vi "3 Axis Step Move.vi"(0 "Reference In":refnum<class "_Controller.lvclass">, 3 "Move":bool, 7 "Error In":errorcluster, 8 "X Steps":string="0", 9 "Direction X":bool=TRUE, 10 "Y Steps":string="0", 11 "Direction Y":bool=TRUE, 12 "Z Steps":string="0", 13 "Direcition Z":bool=TRUE) -> (20 "Reference Out":refnum<class "_Controller.lvclass">, 27 "Error Out":errorcluster)   [LabVIEW 2020]
doc: "Sends commands to the machine to move it in all 3 axes. Default values set at 0 steps, so can be used to only move in 2/3 axes or 1/3 axes. Made up of a series of sub_vi's (in a case structure) to move it in all 3 axis's with their respective inputs being the number of steps it needs to move as well as the direction that motor needs to move in. \n\nArgs:\n\nReference In: Incoming communication (reference) between LabView and the scanning rig controller\nError In: Checks for any errors with the incoming communication (reference)\nX Steps: Number of steps in the X direction\nY Steps: Number of steps in the Y direction\nZ Steps: Number of steps in the Z direction\nDirection X: Direction that the X stepper motor needs to move in\nDirection Y: Direction that the Y stepper motor needs to move in\nDIrection Z: Direction that the Z stepper motor needs to move in\n\nReturns:\n\nReference Out: Output communnication (reference) between LabView and controller\nError Out: Checks for any error with output communication (reference)"
uses:
  <instrlib>/Arcus Ethernet Driver 1.0.0/ArcusEthernetComm/classes/Controller/_Controller.lvclass
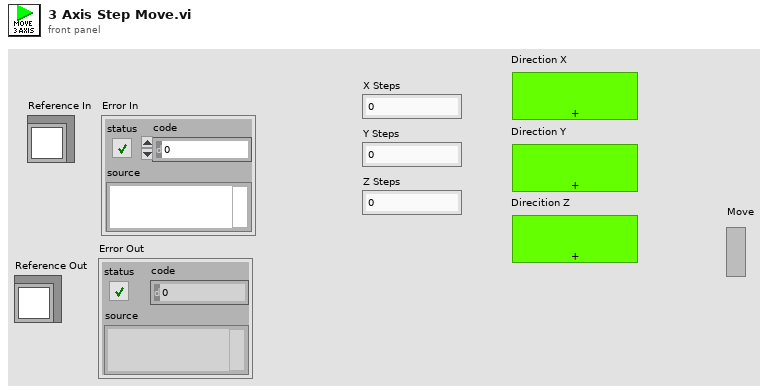
[diagram p1: front panel]
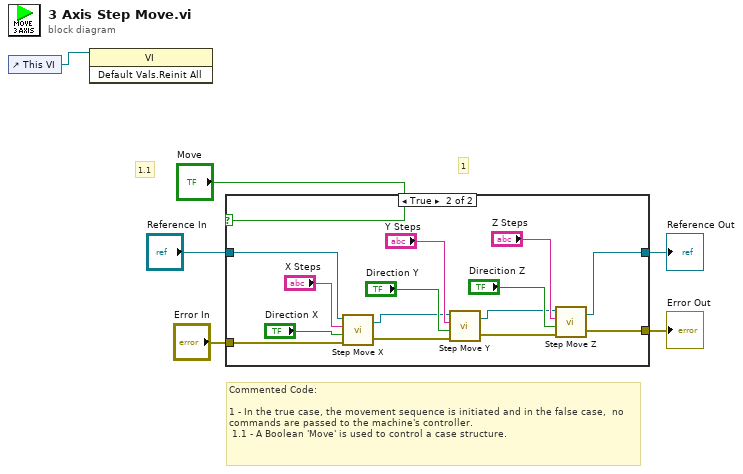
[diagram p0: block diagram]
diagram:
  # "1"
  # "1.1"
  # "Commented Code:\n\n1 - In the true case, the movement sequence is initiated and in the false case,  no commands are passed to the machine's controller.\n 1.1 - A Boolean 'Move' is used to control a case structure."
  n1 = control-ref of="This VI"() -> (w1:refnum<vi>)
  n2 = invoke class="VI" method="Default Vals.Reinit All"(reference=w1) -> ()  [unwired: 2 in, 3 out]
  n3 = case shown="True" "Move" {
    tunnel: "Reference In" -> [w8 w22]
    tunnel: "Error In" -> [w7 w21]
    tunnel: [w8 w12] -> w4
    tunnel: [w7 w11] -> w3
    frame False {
    }
    frame True {
      n4 = call "Step Move X.vi"("Error In"=w21, "Direction"="Direction X", "No. of X Steps"="X Steps", "Reference In"=w22) -> ("Error Out"=w9:errorcluster, "Reference Out"=w14:refnum<class "_Controller.lvclass">)
      n5 = call "Step Move Y.vi"("Error In"=w9, "Direction"="Direction Y", "No. of Y Steps"="Y Steps", "Reference In"=w14) -> ("Error Out"=w10:errorcluster, "Reference Out"=w13:refnum<class "_Controller.lvclass">)
      n6 = call "Step Move Z.vi"("Error In"=w10, "Direction"="Direcition Z", "No. of Z Steps"="Z Steps", "Reference In"=w13) -> ("Error Out"=w11:errorcluster, "Reference Out"=w12:refnum<class "_Controller.lvclass">)
    }
  }
  "Reference Out" <- w4
  "Error Out" <- w3
